vi "Write Stock Trader.vi"(8 "error in (no error)":errorcluster, 10 "Stock Trader":refnum<class "Stock Trader.lvclass">, 11 "Order in":refnum<class "Order.lvclass">) -> (0 "error out":errorcluster, 3 "Order out":refnum<class "Order.lvclass">)   [LabVIEW 2019, in "Order.lvclass"]
doc: "Allows you to initialize the stock trader that acts as an order's reciever"
uses:
  Order.lvclass
  Stock Trader/Stock Trader.lvclass
  Order.lvclass/Order.ctl
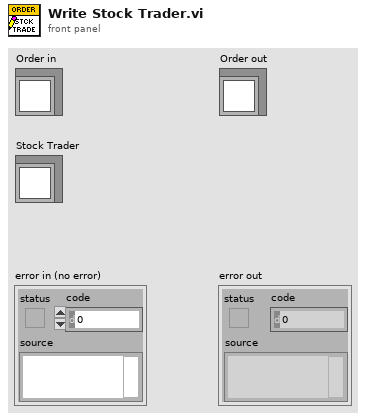
[diagram p1: front panel]
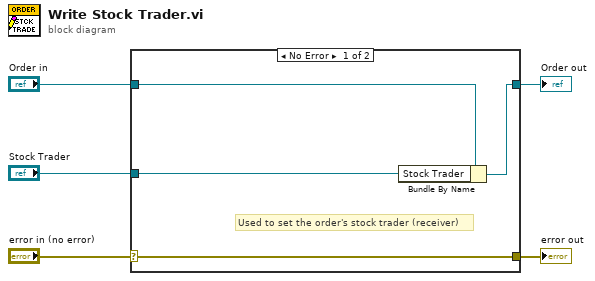
[diagram p0: block diagram]
diagram:
  n1 = case shown="No Error" "error in (no error)" {
    selector: "error in (no error)" -> [w9 w10]
    tunnel: [w9 w10] -> w4
    tunnel: [w7 w11] -> w2
    tunnel: "Order in" -> [w8 w11]
    tunnel: "Stock Trader" -> [w6 _]
    frame No Error {
      # "Used to set the order's stock trader (receiver)"
      n2 = Bundle By Name(cluster=w8, "Stock Trader"=w6) -> (w7:refnum<class "Order.lvclass">)
    }
    frame Error {
    }
  }
  "error out" <- w4
  "Order out" <- w2
